vi "ilemt_globals.vi"() -> ()   [LabVIEW 2024]
uses:
  processing/modulation_info.ctl
  processing/carrier_amplitudes.ctl
  processing/card_carrier_amplitudes.ctl
  calibration/6dof_calibration.ctl
panel:
  out "6DOF Calibration":T1
  in  "Coupling signs":i32[](array[numeric])=[1, -1, -1] min=-1 max=1 step=1
  in  "GUI reference":T2=[[[[0.02387331119477671-0.18792542940648066i, -5.113915405782492e-08+1.477201236518985e-08i, -5.909926197431938e-08+9.545666577928603e-08i], [2.1286570587794595e-09-5.0402429228532664e-08i, -0.07912748753721097-0.17950871296478477i, -1.3336393295260152e-08-2.0138465020580476e-08i], [2.2072236260071987e-08+3.9941466854417906e-08i, 7.554518628716256e-09+2.6635181712975076e-08i, -0.16051353629098078-0.11955944118120924i]], [[0.04447611661980124-0.0022271374618770936i, 1.2261591694496704e-08-6.138375929608728e-08i, -1.1387735087767037e-07+8.338752869683435e-08i], [-7.683639723940697e-09+1.0058220823871729e-07i, 0.04811128784168397-0.0029390541930299128i, -1.7560235231330632e-08-8.652265601942925e-08i], [3.11210525916285e-09+3.808210745168175e-08i, -7.342361599992575e-08+1.38411423615672e-07i, 0.05391763944588081-0.003574818411294752i]]], [[[0.036490720598492926+0.0031504748997741834i, 0.0013698809108581155+0.00011990788393271082i, 0.005331408868789814+0.0004038778874274683i], [-0.001927376717585191+0.0009694701022708568i, 0.05038248918599697-0.025296020831336148i, 4.3742828948548085e-05-6.575941243022743e-05i], [0.004844464386946783-0.007527547985398947i, -0.0013594569088396825+0.0020777067301147017i, -0.07186525116532198+0.1152489228401547i]], [[1.5995302874853427e-05+0.0003089772930155352i, 6.092855117603562e-07+1.1559932110280688e-05i, 2.316791543931251e-06+4.4919033065800296e-05i], [-1.0161603556761576e-06-1.6480630816566404e-05i, 2.7146707073303012e-05+0.000431075740581211i, 5.760250785652257e-08+6.825442859480322e-07i], [4.431803129263396e-06+6.490624248391556e-05i, -1.174220215449416e-06-1.7901057044940623e-05i, -6.594433748534696e-05-0.0009605761484459109i]]]] format="%#_3p"
  out "Source output":T3=[[[0.39991712412028557+0.0004389061145034029i, 3.9477995182648896e-05-0.00021370427071621995i, 4.3868970125876795e-05-1.801567289444482e-05i], [3.2160718284134676e-05-0.0003485529998310377i, 0.3998092930647042+0.0007825109514634835i, 2.9066289166956018e-05-0.00016821381521897282i], [4.447041070486787e-05-0.0002084445665831i, 3.35643782524826e-05-0.0004715169469692911i, 0.3998022671523141+0.0003835728357409047i]], [[0.10000429797260343+1.7832266186313747e-06i, 3.9852830438722545e-07-1.296039228611159e-06i, 3.84597409039583e-07+4.881126203142051e-07i], [3.207922394997762e-07-2.7976416984559625e-06i, 0.09999864705661919+5.096475838982932e-06i, 3.607268904821382e-07-5.243014470180653e-07i], [3.970984058226353e-07-1.7166806248986766e-06i, 3.8616799777759325e-07-3.209680516584786e-06i, 0.10000655291095165-7.426093721638081e-07i]]] format="%#_3p"
  out "Source frequency response":T3=[[[0.05968317538449497-0.4698148755537627i, 0.0732930872824336-0.47831889896803687i, 0.09431406354459475-0.5178417862052147i], [-0.23188208422948645-0.4540136507821202i, -0.1978191640758873-0.44877273057260253i, -0.18847481579426797-0.4805240272268637i], [-0.50937882961812-0.25399185088114096i, -0.4179673739547391-0.2748221776379422i, -0.40128390747244025-0.29889896833054835i]], [[0.44476155056686667-0.022271412976268848i, 0.4814242604799463-0.023912149272769002i, 0.5397475828951473-0.026077028676969295i], [0.4444988965736753-0.027404084961815303i, 0.48111382049307505-0.029390356344307506i, 0.539411552890273-0.032138928091547864i], [0.4443042300124333-0.030434891712612537i, 0.4808998436231261-0.03265598124023235i, 0.5391765615565359-0.03574835625950266i]]] format="%#_3p"
  in  "TCP output connection":refnum<k5>
  in  "Reference amplitudes":T2=[[[[0.023873111550744553-0.1879262838690306i, -3.58536578956542e-08-2.358637043187264e-08i, 3.562026385370723e-08-4.229771289987117e-08i], [-1.1165636529079925e-08-4.7422363279314705e-08i, -0.0791275922079043-0.17950869075430248i, -3.916214574850585e-10+2.1780778299007597e-08i], [-6.839749257508271e-08-1.950152900623281e-08i, 2.836479180701179e-08-5.443184722397909e-09i, -0.16051344136345047-0.11955917661646595i]], [[0.04447616419362632-0.002227172026038178i, 3.3740704730177767e-08+4.049350851484834e-08i, -2.5692927157990318e-09-1.191555445858912e-09i], [-1.834211574609047e-08-5.420421643034033e-08i, 0.0481112768589925-0.0029390137172910584i, 6.906388682852483e-08+7.575659695975117e-08i], [-3.672700693372587e-08+8.573538658350061e-09i, 3.318795525576407e-09+3.6519606645564015e-09i, 0.05391750204276394-0.0035748429030597302i]]], [[[0.0364908855431503+0.0031504080385310806i, 0.0013698683586229566+0.00011990104025593958i, 0.005331511779096097+0.00040393827607082794i], [-0.001927459645915089+0.0009694376935085788i, 0.05038248677785455-0.025296001287764124i, 4.379667308327534e-05-6.567966649612123e-05i], [0.004844522332222083-0.007527673549449875i, -0.0013593229864157057+0.002077668322084983i, -0.07186514340494729+0.11524875168058052i]], [[1.6015148573742124e-05+0.0003089085978094754i, 6.39812835343047e-07+1.158938843541178e-05i, 2.299328909500673e-06+4.486287484386544e-05i], [-1.0371617895174975e-06-1.6557740189737855e-05i, 2.7180888423383594e-05+0.00043116591879711045i, 7.787505158470277e-08+7.343229374258908e-07i], [4.398945095918059e-06+6.489502538901468e-05i, -1.2085704809037543e-06-1.7891520277375576e-05i, -6.592496668152256e-05-0.0009606768385914297i]]]] format="%#_3p"
  in  "Carrier amplitudes":T2=[[[[-0.20547792043209226-0.05502943856352568i, 2.0436757981922964e-05+2.4746833152413713e-06i, 2.2672098115323675e-05+2.629033574994465e-06i], [1.2144717257371075e-05-4.13724290940741e-06i, -0.14655644652404018+0.039656827776363875i, 5.552395999999099e-06-2.970007202856076e-06i], [7.480505757312579e-06-7.287068968716073e-06i, 2.7414579122191085e-06-3.604565275485208e-06i, -0.09199418701864949+0.08897475046271823i]], [[0.09124870692300698-0.15737469991731665i, -1.4005060518503155e-05+7.224773509231025e-05i, -1.3551405332751143e-05+7.618236190666783e-05i], [5.564021637520272e-07+4.811437162437222e-05i, 0.0673340984306771-0.1487717792617868i, 5.9823453563539896e-06+4.431827771148551e-05i], [4.28647709472648e-06+5.3755891132260515e-05i, 1.1774247187831415e-05+4.428661259267218e-05i, 0.06616726428364414-0.1626927804601966i]]], [[[-0.024646227324105225+0.14588928877147012i, 0.008146924678786492-0.04732594100818745i, 0.004654222563486155-0.02768135782961336i], [-0.004164007704859315-0.009165749798000822i, 0.028517033295292916+0.061095278115674403i, -0.000318867252001585-0.00031544189325922447i], [-0.03025104780254181-0.015639398032304748i, 0.005475445706818961+0.00403665175711173i, 0.09967462565752472+0.045601054018610906i]], [[-0.003255555555159672-0.0017493408885658466i, 0.0010622703191949107+0.0005710707263271102i, 0.0006286044983085689+0.0003381219213888351i], [0.00021091331509259808+8.669718932974928e-05i, -0.0012908146116934237-0.0005360584709089646i, -6.1850936260488635e-06-2.4526401815922687e-06i], [0.0005015406058025835+0.00018663227842703243i, -0.000133717568862518-4.996647989133334e-05i, -0.0014464988279219398-0.0005404549892277387i]]]] format="%#_3p"
  in  "Modulation info":T4={"Fs full"=0.0, "Fs high"=0.0, "Fs low"=0.0, "Read size"=5000, "FFT size low"=5000, "df low"=5000.0, "High carriers"=[], "Low carriers"=[], "Hi channels at low"=[7]} {"Hi channels at low" min=0 step=1; "Low carriers" format="%#_6p"; "High carriers" format="%#_6p"}
  in  "TCP input connection":refnum<k5>
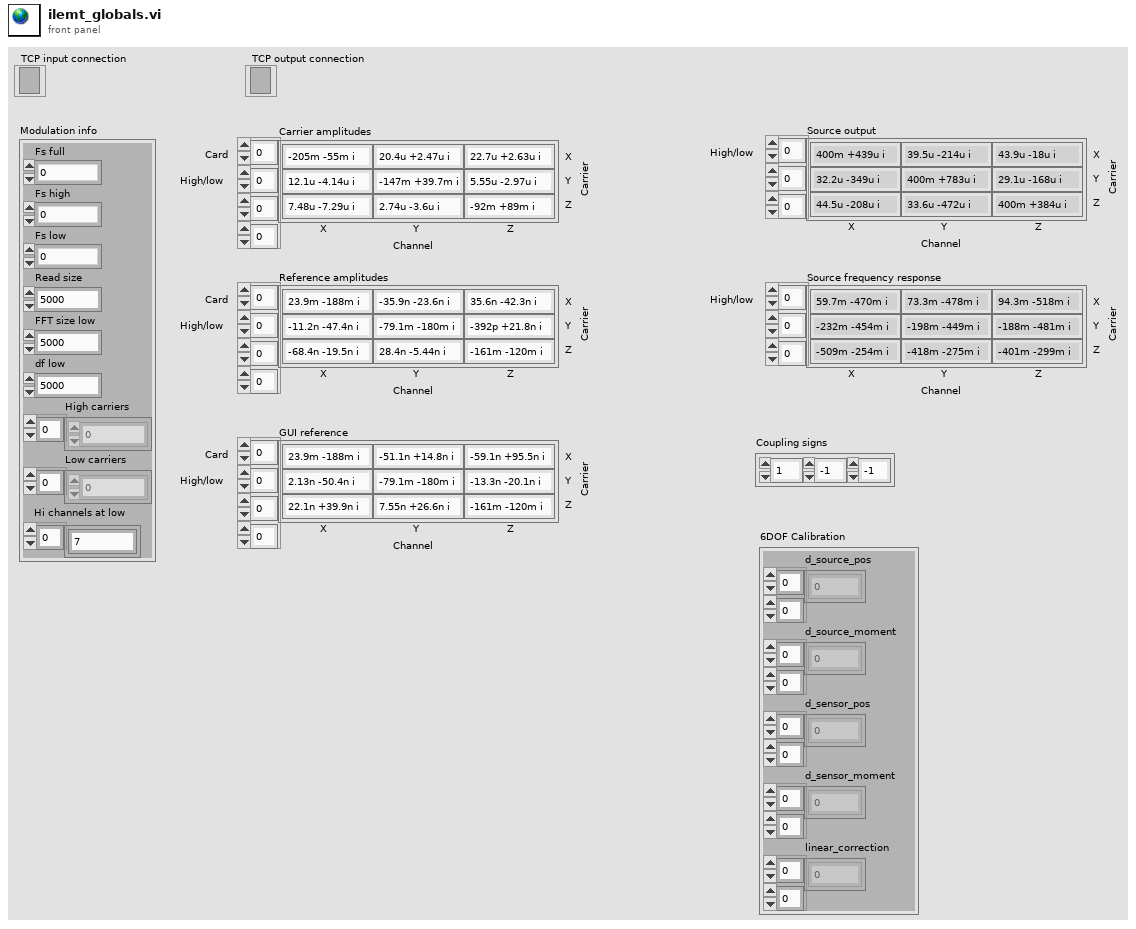
[diagram p1: front panel]
types:
  T1 = typedef "6dof_calibration.ctl" = cluster{"d_source_pos":dbl[][], "d_source_moment":dbl[][], "d_sensor_pos":dbl[][], "d_sensor_moment":dbl[][], "linear_correction":dbl[][]}
  T2 = typedef "carrier_amplitudes.ctl" = cdb[][][][]
  T3 = typedef "card_carrier_amplitudes.ctl" = cdb[][][]
  T4 = typedef "modulation_info.ctl" = cluster{"Fs full":dbl, "Fs high":dbl, "Fs low":dbl, "Read size":i32, "FFT size low":i32, "df low":dbl, "High carriers":dbl[], "Low carriers":dbl[], "Hi channels at low":i32[]}
diagram:
